vi "getLoss.vi"(8 "error in (no error)":errorcluster, 11 "Inst.AH2500 in":refnum<class "Inst.AH2500.lvclass">) -> (0 "error out":errorcluster, 2 "Loss (S)":dbl, 3 "Inst.AH2500 out":refnum<class "Inst.AH2500.lvclass">)   [LabVIEW 2019, in "Inst.AH2500.lvclass"]
uses:
  Inst.AH2500.lvclass
  C:/Program Files/National Instruments/LabVIEW 2019/user.lib/LevyLab/Instrument Framework/Instrument/Instrument.lvclass
  Typedefs/Inst.AH2500.Commands--Enum.ctl
  Typedefs/Inst.AH2500.getAll--Cluster.ctl
  991804cd-2d63-4689-a149-8f7b841441b7.vi/57c753f5-5212-453e-972d-aea4c9ef8994.vi
  991804cd-2d63-4689-a149-8f7b841441b7.vi/57c753f5-5212-453e-972d-aea4c9ef8994.vi/d35fc7f8-dffb-483e-877e-d52e694eda9f.vi
  991804cd-2d63-4689-a149-8f7b841441b7.vi/57c753f5-5212-453e-972d-aea4c9ef8994.vi/55c84151-b5b2-4f55-839f-365cf900fbe5.vi
  <vilib>/Utility/Data Type/Get Type Information.vi
  <vilib>/JDP Science/JSONtext/JSON text to Variant.vi
  <vilib>/JDP Science/JSONtext/LVClass Serializer/JSONtext LVClass Serializer.lvclass
  <userlib>/LevyLab/Instrument Framework/Instrument/Instrument.lvclass
  a4717982-6b33-437d-a08c-f86142bf163a.vi
  C:/Program Files/National Instruments/LabVIEW 2019/user.lib/LevyLab/Instrument Framework/Instrument Types/CBridge/Instrument.CBridge.lvclass
  C:/Program Files/National Instruments/LabVIEW 2019/vi.lib/JKI/JKI SMO/SMO/SMO.lvclass
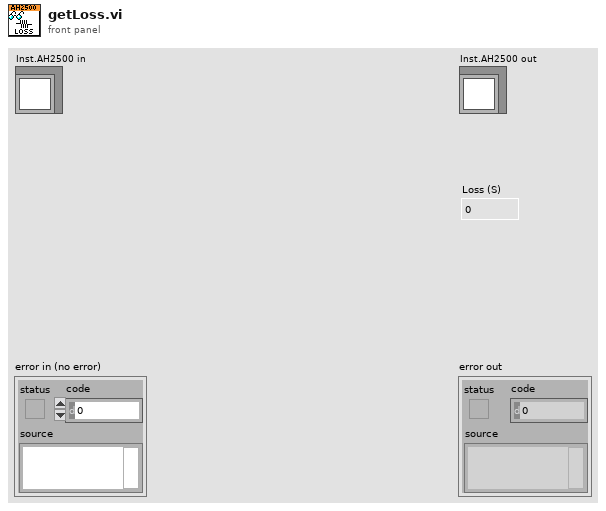
[diagram p1: front panel]
types:
  T1 = typedef "Inst.AH2500.lvclass/Inst.AH2500.getAll--Cluster.ctl" = cluster{"capacitance (pF)":dbl, "loss (nS)":dbl, "Vexc (V)":dbl}
  T2 = typedef "Inst.AH2500.lvclass/Inst.AH2500.Commands--Enum.ctl" = enum16{"getCapacitance", "getLoss", "getExcitation"}
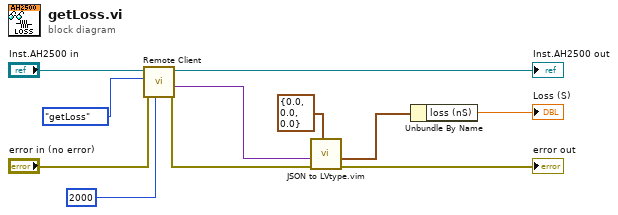
[diagram p0: block diagram]
diagram:
  n1 = call <userlib>:"Remote Client.vi"("timeout (ms) [500]"=2000 ("timeout (ms) test string"), "error in (no error)"="error in (no error)", "Command in"=Inst.AH2500.Commands--Enum."getLoss" ("Commands"), "Instrument in"="Inst.AH2500 in") -> ("error out"=w2:errorcluster, "Data out"=w4:variant, "Instrument out"=→"Inst.AH2500 out":refnum<class "Inst.AH2500.lvclass">)  [unwired: 4 in, 1 out]
  n2 = call "JSON to LVtype.vim"("type"=T1 {"capacitance (pF)"=0.0, "loss (nS)"=0.0, "Vexc (V)"=0.0} ("getAll"), "error in (no error)"=w2, "JSON Data in"=w4) -> ("error out"=→"error out":errorcluster, "Data out"=w6:T1)  [unwired: 7 in]
  n3 = Unbundle By Name(w6) -> ("loss (nS)"=→"Loss (S)":dbl)
